vi "Send scan2d_perform_scan.vi"(7 "Message Priority (Normal)":T3=enum."Normal", 8 "error in (no error)":errorcluster, 10 "scan-2d-settings":T1, 11 "Message Enqueuer":refnum<class "Message Enqueuer.lvclass">) -> (0 "error out":errorcluster, 3 "Message Enqueuer out":refnum<class "Message Enqueuer.lvclass">)   [LabVIEW 2015, in "scan2d_perform_scan Msg.lvclass"]
doc: "This VI sends the message to an actor."
uses:
  scan2d_perform_scan Msg.lvclass
  <vilib>/ActorFramework/Message Enqueuer/Message Enqueuer.lvclass
  <vilib>/ActorFramework/Message Enqueuer/Message Priority.ctl
  2d_scan/scan_2d_settings.ctl
  Scan/scan_record.ctl
  scan2d_perform_scan Msg.lvclass/scan2d_perform_scan Msg.ctl
  <vilib>/ActorFramework/Message Enqueuer/Message Enqueuer.lvclass/Message Enqueuer.ctl
  <vilib>/ActorFramework/Message Priority Queue/Priority Enqueue.vi
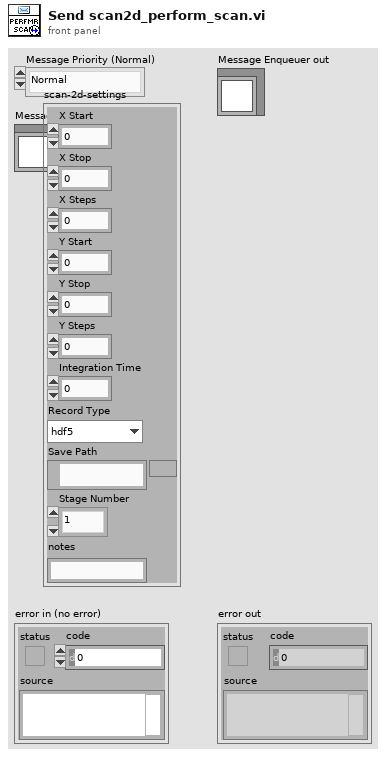
[diagram p1: front panel]
types:
  T1 = typedef "scan_2d_settings.ctl" = cluster{"X Start":dbl, "X Stop":dbl, "X Steps":u32, "Y Start":dbl, "Y Stop":dbl, "Y Steps":u32, "Integration Time":dbl, "Record Type":T2, "Save Path":path, "Stage Number":enum16{"1", "2"}, "notes":string}
  T2 = typedef "scan_record.ctl" = enum16{"hdf5", "legacy", "None"}
  T3 = typedef "Actor Framework.lvlib/Message Enqueuer.lvclass/Message Priority.ctl" = enum16{"Low", "Normal", "High"}
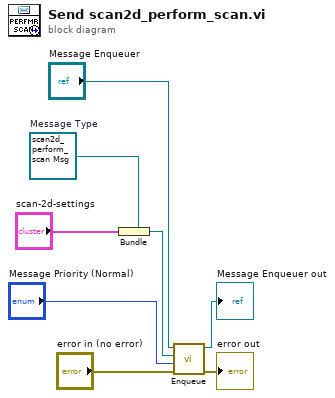
[diagram p0: block diagram]
diagram:
  w5 = refnum<class "scan2d_perform_scan Msg.lvclass"> refnum  # Message Type
  n1 = Bundle(cluster=w5, "scan-2d-settings") -> (w4:refnum<class "scan2d_perform_scan Msg.lvclass">)
  n2 = call <vilib>:"Enqueue.vi"("error in (no error)"="error in (no error)", "Message Priority (Normal)"="Message Priority (Normal)", "Message"=w4, "Message Enqueuer in"="Message Enqueuer") -> ("error out"=→"error out":errorcluster, "Message Enqueuer out"=→"Message Enqueuer out":refnum<class "Message Enqueuer.lvclass">)  [unwired: 6 in]
